vi "Main Time To Freq.vi"(1 "Main Time":u16) -> (0 "Frequency (Hz)":dbl)   [LabVIEW 2019]
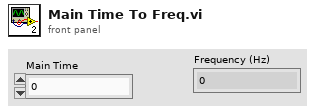
[diagram p1: front panel]
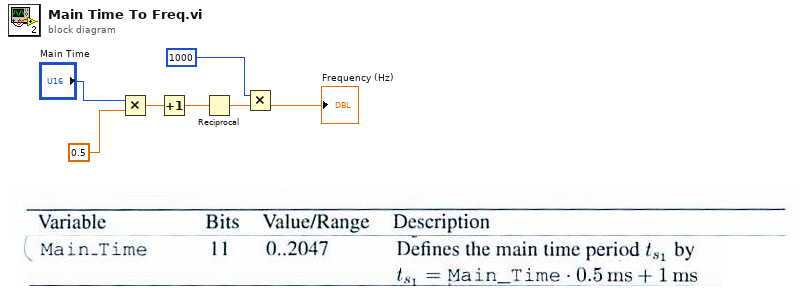
[diagram p0: block diagram]
diagram:
  n1 = Multiply(x="Main Time", y=0.5) -> (x*y=w5:dbl)
  n2 = Increment(x=w5) -> (x+1=w3:dbl)
  n3 = Reciprocal(x=w3) -> (1/x=w4:dbl)
  n4 = Multiply(x=1000, y=w4) -> (x*y=→"Frequency (Hz)":dbl)
